vi "Get Spec Info.vi"(0 "COM Port In":refnum<visa-resource-name>, 1 "error out":errorcluster caption="error in") -> (2 "COM Port out":refnum<visa-resource-name>, 3 "Spec Info":cluster{string, "read buffer":string}, 4 "OK":bool, 5 "error out 2":errorcluster caption="error out")   [LabVIEW 2015]
doc: "This command receives the specified power and the wavelength of the connected device.\nThese specifications are for informative use only."
panel:
  out "Numerisch":i32
  out "Wavelength":string
  out "Spec Power":string
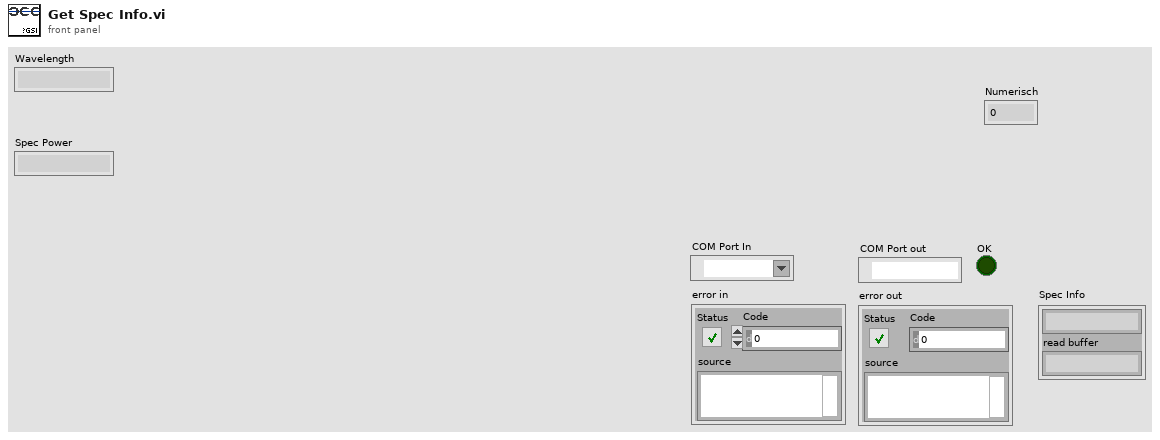
[diagram p1: front panel]
types:
  T1 = cluster{"read buffer":string, "read buffer":string}
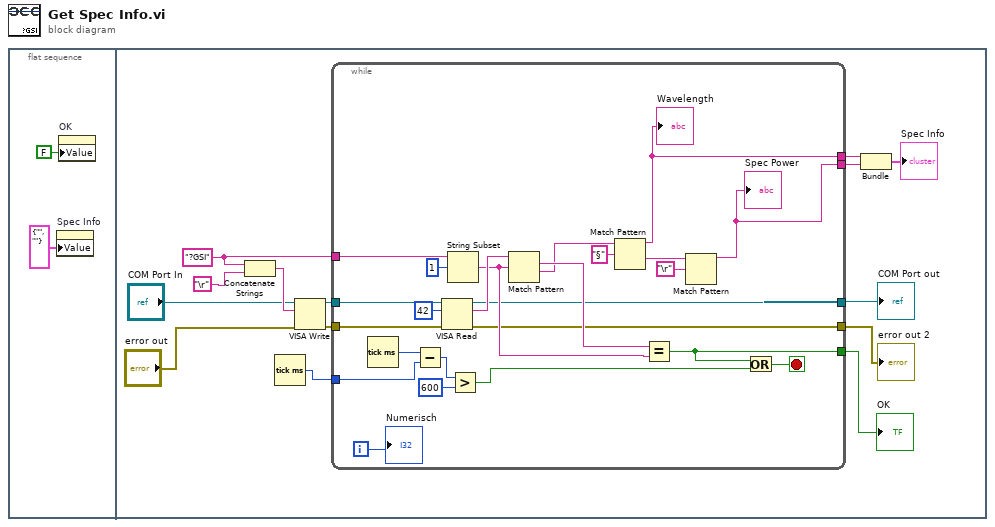
[diagram p0: block diagram]
diagram:
  n1 = flat-sequence {
    frame #0 {
      n2 = property on="Spec Info" class="Clust (strict)"("Value"=cluster{string, "read buffer":string} {"", "read buffer"=""} ("Spec Info")) -> ()  [unwired: 2 in, 2 out]
      n3 = property on="OK" class="Bool (strict)"("Value"=FALSE ("OK")) -> ()  [unwired: 2 in, 2 out]
    }
    frame #1 {
      w7 = "?GSI" ("Schreibpuffer")
      n4 = Concatenate Strings(w7, "\r") -> (w11:string)
      n5 = Tick Count (ms)() -> (millisecond timer value=w3:u32)
      n6 = VISA Write(VISA resource name="COM Port In", write buffer=w11, error in (no error)="error out") -> (VISA resource name out=w9:refnum<visa-resource-name>, error out=w8:errorcluster)  [unwired: 1 out]
      n7 = while {
        tunnel: [w29] -> w16
        tunnel: [w33] -> w13
        tunnel: [w32] -> w12
        tunnel: [w31] -> w15
        tunnel: w9 -> [w24]
        tunnel: w8 -> [w27]
        tunnel: w7 -> [w26]
        tunnel: [w25] -> w4
        tunnel: w3 -> [w20]
        i -> [w18]
        stop <- w30 stop-if-true
        n8 = Tick Count (ms)() -> (millisecond timer value=w21:u32)
        n9 = Subtract(x=w21, y=w20) -> (x-y=w22:u32)
        n10 = VISA Read(VISA resource name=w24, byte count=u32 42 ("Byte-Anzahl"), error in (no error)=w27) -> (VISA resource name out=w33:refnum<visa-resource-name>, read buffer=w38:string, error out=w32:errorcluster)  [unwired: 1 out]
        n11 = String Subset(string=w26, offset (0)=1 ("Offset (0)")) -> (substring=w34:string)  [unwired: 1 in]
        n12 = Greater?(x=w22, y=u32 600) -> (0:w19:bool)
        n13 = Match Pattern(string=w38, regular expression=w34) -> (match substring=w37:string, after substring=w36:string)  [unwired: 1 in, 2 out]
        n14 = Match Pattern(string=w36, regular expression="§" ("Nach String/Zeichen suchen (-)")) -> (before substring=w29:string, after substring=w28:string)  [unwired: 1 in, 2 out]
        "Wavelength" <- w29
        n15 = Equal?(x=w37, y=w34) -> (x = y?=w25:bool)
        n16 = Match Pattern(string=w28, regular expression="\r") -> (before substring=w31:string)  [unwired: 1 in, 3 out]
        "Spec Power" <- w31
        n17 = Or(x=w25, y=w19) -> (x .or. y?=w30:bool)
        "Numerisch" <- w18
      }
      "OK" <- w4
      "COM Port out" <- w13
      "error out 2" <- w12
      n18 = Bundle("read buffer"=w16, "read buffer"=w15) -> (→"Spec Info":T1)  [unwired: 1 in]
    }
  }
